vi "UHR-Fleezers Control (host) -Mau_stepping.vi"(0 "Tab Control":T5(tab)) -> ()   [LabVIEW 2013] (continued)
            n684 = local read "Green FB On/Off"() -> (w1119:bool)
            n685 = Equal?(x=w1122, y=enum32{"Laser ON", "Laser OFF", "Interlace"}."Interlace") -> (x = y?=w1120:bool)
            n686 = And(x=w1120, y=w1119) -> (x .and. y?=w1118:bool)
          }
        }
        n687 = xnode "Read/Write Control"("FPGA VI Reference In"=w1115, "error in"=w1113, "Operating Mode"=w1110, "Operating Mode 2"=w1110, "Green FB On/Off"=w1109) -> ("error out"=w1114:errorcluster)  [unwired: 1 out]
      }
      event "- phase (APD 1 Gate)", "+ phase (APD 1 Gate)": Value Change {
        n688 = event-data() -> ()  [unwired: 7 out]
        n689 = local read "Phase Adj. (APD 1 Gate)"() -> (w1123:i16)
        n690 = Negate(x=w1123) -> (-x=w1131:i16)
        n691 = Select(t=w1131, s="- phase (APD 1 Gate)", f=w1123) -> (s? t:f=w1130:i16)
        n692 = Or(x="- phase (APD 1 Gate)", y="+ phase (APD 1 Gate)") -> (x .or. y?=w1126:bool)
        n693 = xnode "Read/Write Control"("FPGA VI Reference In"=w1133, "error in"=w1132, "Phase count adjustment (APD 1 Gate)"=w1130) -> ("FPGA VI Reference Out"=w1128:T19, "error out"=w1129:errorcluster)
        n694 = xnode "Read/Write Control"("FPGA VI Reference In"=w1128, "error in"=w1129, "+ phase (APD 1 Gate)"=w1126) -> ("error out"=w1127:errorcluster)  [unwired: 1 out]
      }
      event "+ phase (APD 2 Gate)", "- phase (APD 2 Gate)": Value Change {
        n695 = event-data() -> ()  [unwired: 7 out]
        n696 = local read "Phase Adj. (APD 2 Gate)"() -> (w1134:i16)
        n697 = Negate(x=w1134) -> (-x=w1142:i16)
        n698 = Select(t=w1142, s="- phase (APD 2 Gate)", f=w1134) -> (s? t:f=w1141:i16)
        n699 = Or(x="- phase (APD 2 Gate)", y="+ phase (APD 2 Gate)") -> (x .or. y?=w1137:bool)
        n700 = xnode "Read/Write Control"("FPGA VI Reference In"=w1144, "error in"=w1143, "Phase count adjustment (APD 2 Gate)"=w1141) -> ("FPGA VI Reference Out"=w1139:T19, "error out"=w1140:errorcluster)
        n701 = xnode "Read/Write Control"("FPGA VI Reference In"=w1139, "error in"=w1140, "+ phase (APD 2 Gate)"=w1137) -> ("error out"=w1138:errorcluster)  [unwired: 1 out]
      }
      event "Phase Adj. (APD Acq)", "+ phase (APD Acq)", "- phase (APD Acq)": Value Change {
        n702 = event-data() -> ()  [unwired: 7 out]
        n703 = local read "Phase Adj. (APD Acq)"() -> (w1147:i16)
        n704 = Negate(x=w1147) -> (-x=w1153:i16)
        n705 = Select(t=w1153, s="+ phase (APD Acq)", f=w1147) -> (s? t:f=w1152:i16)
        n706 = Or(x="+ phase (APD Acq)", y="- phase (APD Acq)") -> (x .or. y?=w1148:bool)
        n707 = xnode "Read/Write Control"("FPGA VI Reference In"=w1155, "error in"=w1154, "Phase Count Adjustment (APD Acq)"=w1152) -> ("FPGA VI Reference Out"=w1150:T19, "error out"=w1151:errorcluster)
        n708 = xnode "Read/Write Control"("FPGA VI Reference In"=w1150, "error in"=w1151, "+ phase (APD Acq)"=w1148) -> ("error out"=w1149:errorcluster)  [unwired: 1 out]
      }
      event "Phase adj. (GI)", "+ phase (GI)", "- phase (GI)": Value Change {
        n709 = event-data() -> ()  [unwired: 7 out]
        n710 = Negate(x="Phase adj. (GI)") -> (-x=w1164:i16)
        n711 = Select(t=w1164, s="+ phase (GI)", f="Phase adj. (GI)") -> (s? t:f=w1163:i16)
        n712 = Or(x="+ phase (GI)", y="- phase (GI)") -> (x .or. y?=w1159:bool)
        n713 = xnode "Read/Write Control"("FPGA VI Reference In"=w1166, "error in"=w1165, "Phase count adjustment (GI)"=w1163) -> ("FPGA VI Reference Out"=w1161:T19, "error out"=w1162:errorcluster)
        n714 = xnode "Read/Write Control"("FPGA VI Reference In"=w1161, "error in"=w1162, "+ phase (GI)"=w1159) -> ("error out"=w1160:errorcluster)  [unwired: 1 out]
      }
      event "Phase adj. (GI) 2", "+ phase (GI) 2", "- phase (GI) 2": Value Change {
        n715 = event-data() -> ()  [unwired: 7 out]
        n716 = Negate(x="Phase adj. (GI) 2") -> (-x=w1175:i16)
        n717 = Select(t=w1175, s="+ phase (GI) 2", f="Phase adj. (GI) 2") -> (s? t:f=w1174:i16)
        n718 = Or(x="+ phase (GI) 2", y="- phase (GI) 2") -> (x .or. y?=w1170:bool)
        n719 = xnode "Read/Write Control"("FPGA VI Reference In"=w1177, "error in"=w1176, "Phase count adjustment (GI) 2"=w1174) -> ("FPGA VI Reference Out"=w1172:T19, "error out"=w1173:errorcluster)
        n720 = xnode "Read/Write Control"("FPGA VI Reference In"=w1172, "error in"=w1173, "+ phase (GI) 2"=w1170) -> ("error out"=w1171:errorcluster)  [unwired: 1 out]
      }
      event "Phase adj. (Green FB)", "- phase (Green FB)", "+ phase (Green FB)": Value Change {
        n721 = event-data() -> ()  [unwired: 7 out]
        n722 = Negate(x="Phase adj. (Green FB)") -> (-x=w1186:i16)
        n723 = Select(t=w1186, s="+ phase (Green FB)", f="Phase adj. (Green FB)") -> (s? t:f=w1185:i16)
        n724 = Or(x="+ phase (Green FB)", y="- phase (Green FB)") -> (x .or. y?=w1181:bool)
        n725 = xnode "Read/Write Control"("FPGA VI Reference In"=w1188, "error in"=w1187, "Phase count adjustment (Green FB)"=w1185) -> ("FPGA VI Reference Out"=w1183:T19, "error out"=w1184:errorcluster)
        n726 = xnode "Read/Write Control"("FPGA VI Reference In"=w1183, "error in"=w1184, "+ phase (Green FB)"=w1181) -> ("error out"=w1182:errorcluster)  [unwired: 1 out]
      }
      event "Invert APD Gate", "APD Gate ON Count", "APD Gate OFF Count", "APD Gate", "APD Integration Time (s)", "APD 1 AO Mult.", "APD 2 AO Mult.": Value Change {
        n727 = event-data() -> ()  [unwired: 7 out]
        n728 = local read "APD Integration Time (s)"() -> (w1189:dbl)
        n729 = local read "APD Gate ON Count"() -> (w1202:u32)
        n730 = local read "APD Gate OFF Count"() -> (w1201:u32)
        n731 = local read "Invert APD Gate"() -> (w1203:bool)
        n732 = local read "APD Gate"() -> (w1200:enum32{"ON", "OFF", "Interlace"})
        n733 = Multiply(x=w1189, y=40000000.0) -> (x*y=w1198:dbl)
        n734 = Reciprocal(x=w1189) -> (1/x=→"APD Acq Rate (Hz)":dbl)
        n735 = To Unsigned Long Integer(number=w1198) -> (unsigned 32bit integer=w1197:u32)
        n736 = local read "DMA Update Period (s)"() -> (w1190:dbl)
        n737 = Divide(x=w1190, y=w1189) -> (x/y=w1193:dbl)
        n738 = local read "APD 1 AO Mult."() -> (w1195:i16)
        n739 = local read "APD 2 AO Mult."() -> (w1194:i16)
        n740 = Multiply(x=2.0, y=w1193) -> (x*y=w1192:dbl)
        n741 = local write "APD Samples/FIFO Acq."(w1193) -> ()
        n742 = local write "APD Elements/DMA read"(w1192) -> ()
        n743 = xnode "Read/Write Control"("FPGA VI Reference In"=w1206, "error in"=w1205, "Invert APD Gate"=w1203, "APD Gate ON Count"=w1202, "APD Gate OFF Count"=w1201, "APD Acq Rate Count"=w1197, "APD Gate Operating Mode"=w1200, "APD 1 AO scale factor"=w1195, "APD 2 AO scale factor"=w1194) -> ("error out"=w1204:errorcluster)  [unwired: 1 out]
      }
      event "GI Frequency, ON count", "Green FB Count", "GI Frequency, OFF count": Value Change {
        n744 = event-data() -> ()  [unwired: 7 out]
        n745 = xnode "Read/Write Control"("FPGA VI Reference In"=w1212, "error in"=w1210, "Green interlace ON count"="GI Frequency, ON count", "Green interlace OFF count"="GI Frequency, OFF count", "Green interlace ON count 2"="GI Frequency, ON count", "Green interlace OFF count 2"="GI Frequency, OFF count", "Green FB Count"="Green FB Count") -> ("error out"=w1211:errorcluster)  [unwired: 1 out]
      }
      event "Number of F/B Scans (AOD)", "Scan Speed (nm/s)", "Scan BD", "Initial delta (MHz)", "Step Size (nm)", "Scan Range (nm)": Value Change {
        w1274 = 123.0  # AOM cal (nm/MHz)
        n746 = event-data() -> ()  [unwired: 7 out]
        n747 = local read "BD 1 Frequency 1 (MHz)"() -> (w1257:dbl)
        n748 = local read "AOM X Cal (nm/MHz)"() -> (w1249:dbl)
        n749 = local read "X RF Frequency Limits (MHz)"() -> (w1261:T16)
        n750 = local read "Y RF Frequency Limits (MHz)"() -> (w1258:T16)
        n751 = local read "BD 2 Frequency 1 (MHz)"() -> (w1263:dbl)
        n752 = Negate(x="Scan Range (nm)") -> (-x=w1227:dbl)
        n753 = Divide(x=w1227, y=w1249) -> (x/y=w1231:dbl)
        n754 = Select(t=w1261, s="Scan BD", f=w1258) -> (s? t:f=w1260:T16)
        n755 = Select(t=w1257, s="Scan BD", f=w1263) -> (s? t:f=w1262:dbl)
        n756 = Unbundle By Name(w1260) -> ("Maximum"=w1269:dbl, "Minimum"=w1268:dbl)
        n757 = Add(x=w1231, y=w1262) -> (x+y=w1266:dbl)
        n758 = Divide(x=w1227, y="Step Size (nm)") -> (x/y=w1246:dbl)
        n759 = Divide(x="Step Size (nm)", y=w1249) -> (x/y=w1255:dbl)
        n760 = Absolute Value(x=w1246) -> (abs(x)=w1230:dbl)
        n761 = Sign(1:w1227) -> (0:w1228:dbl)
        n762 = In Range and Coerce(upper limit=w1269, x=w1266, lower limit=w1268) -> (coerced(x)=w1265:dbl, In Range?=w1267:bool)
        n763 = To Unsigned Quad Integer(1:w1230) -> (0:w1245:u64)
        "Scan steps (AOD)" <- w1245
        n764 = call "IR AOM freq to word.vi"("Frequency In (MHz)"=w1255) -> ("Frequency Word Out (double)"=w1252:dbl)
        n765 = Multiply(x=w1228, y=w1252) -> (x*y=w1229:dbl)
        n766 = Subtract(x=w1266, y=w1265) -> (x-y=w1264:dbl)
        n767 = To Quad Integer(1:w1229) -> (0:w1251:i64)
        "Incr. int (AOD)" <- w1251
        n768 = Subtract(x=w1231, y=w1264) -> (x-y=w1250:dbl)
        "Scan Range (MHz)" <- w1250
        n769 = Select(t=w1231, s=w1267, f=w1250) -> (s? t:f=w1270:dbl)
        n770 = Multiply(x=w1250, y=w1249) -> (x*y=w1248:dbl)
        n771 = Decrement(x=w1245) -> (x-1=w1298:u64)
        n772 = Negate(x=w1248) -> (-x=w1244:dbl)
        n773 = local write "Scan Range (nm)"(w1244) -> ()
        n774 = Divide(x=w1270, y=w1298) -> (x/y=w1254:dbl)
        "Scan Increment (MHz)" <- w1254
        n775 = call "IR AOM freq to word.vi"("Frequency In (MHz)"=w1254) -> ("Frequency Word Out (double)"=w1253:dbl)
        n776 = Divide(x="Step Size (nm)", y="Scan Speed (nm/s)") -> (x/y=w1241:dbl)
        n777 = To Quad Integer(1:w1253) -> ()  [unwired: 1 out]
        n778 = local read "Number Interlace Sets"() -> (w1225:u8)
        n779 = local read "AI Count (ticks)"() -> (w1226:u32)
        n780 = local read "Total Counts (ticks)"() -> (w1224:u32)
        n781 = local read "# Samples/trap"() -> (w1256:u32)
        n782 = Multiply(x=w1226, y=w1225) -> (x*y=w1223:u32)
        n783 = Divide(x=w1224, y=w1223) -> (x/y=w1222:dbl)
        n784 = Select(t=w1257, s="Scan BD", f=w1263) -> (s? t:f=w1295:dbl)
        "Initial freq. (MHz)" <- w1295
        n785 = Add(x=w1270, y=w1295) -> (x+y=→"Final freq. (MHz)":dbl)
        n786 = Divide(x=w1224, y=40000000.0) -> (x/y=w1240:dbl)
        n787 = Divide(x=w1241, y=w1240) -> (x/y=w1239:dbl)
        n788 = To Unsigned Quad Integer(1:w1239) -> (0:w1214:u64)
        n789 = Quotient & Remainder(x=w1214, y=u64 2) -> (x-y*floor(x/y)=w1218:u64)  [unwired: 1 out]
        n790 = Equal?(x=w1218, y=u64 0) -> (x = y?=w1216:bool)
        n791 = Decrement(x=w1214) -> (x-1=w1215:u64)
        n792 = Select(t=w1214, s=w1216, f=w1215) -> (s? t:f=w1213:u64)
        "Cycles/step (AOD)" <- w1213
        n793 = xnode "Read/Write Control"("FPGA VI Reference In"=w1306, "error in"=w1305, "Scan steps"=w1245, "Number of scans"="Number of F/B Scans (AOD)", "Cycles per step"=w1213, "Scan freq.  increment"=w1251, "Scan BD"="Scan BD") -> ("error out"=w1304:errorcluster)  [unwired: 1 out]
        n794 = Multiply(x=w1245, y=w1213) -> (x*y=w1299:u64)
        n795 = Multiply(x=w1299, y=u64 2) -> (x*y=w1221:u64)
        n796 = Multiply(x=w1222, y=w1221) -> (x*y=w1220:dbl)
        "Data points/scan (f/b)" <- w1220
        n797 = Multiply(x=w1220, y="Number of F/B Scans (AOD)") -> (x*y=w1302:dbl)
        "Data points/scans" <- w1302
        n798 = Divide(x=w1302, y=w1256) -> (x/y=→"N sets should be saved":dbl)
        n799 = Multiply(x=w1299, y=w1240) -> (x*y=w1238:dbl)
        "Time/Scan (s) (AOD)" <- w1238
        n800 = Select(t=w1270, s="Scan BD", f=0.0) -> (s? t:f=w1296:dbl)
        n801 = Select(t=0.0, s="Scan BD", f=w1270) -> (s? t:f=w1292:dbl)
        n802 = local read "BD 2 Frequency 2 (MHz)"() -> (w1288:dbl)
        n803 = local read "BD 1 Frequency 2 (MHz)"() -> (w1291:dbl)
        n804 = Add(x=w1292, y=w1263) -> (x+y=w1289:dbl)
        n805 = Add(x=w1257, y=w1296) -> (x+y=w1290:dbl)
        n806 = Multiply(x=w1238, y=2.0) -> (x*y=w1237:dbl)
        n807 = Multiply(x=w1237, y="Number of F/B Scans (AOD)") -> (x*y=w1234:dbl)
        n808 = Divide(x=w1234, y=60.0) -> (x/y=→"Time to Finish All (min)":dbl)
        n809 = Add(x="Trap 2 Bead Size (nm)", y="Trap 1 Bead Size (nm)") -> (x+y=w1278:dbl)
        n810 = local read "Initial delta (MHz)"() -> (w1275:dbl)
        n811 = Divide(x=w1278, y=2.0) -> (x/y=w1272:dbl)
        n812 = Subtract(x=w1289, y=w1288) -> (x-y=w1286:dbl)
        n813 = Subtract(x=w1290, y=w1291) -> (x-y=w1287:dbl)
        n814 = Square(x=w1286) -> (x^2=w1285:dbl)
        n815 = Square(x=w1287) -> (x^2=w1284:dbl)
        n816 = Add(x=w1284, y=w1285) -> (x+y=w1283:dbl)
        n817 = Square Root(x=w1283) -> (sqrt(x)=w1282:dbl)
        "Final delta (MHz)" <- w1282
        n818 = Multiply(x=w1274, y=w1282) -> (x*y=w1281:dbl)
        n819 = Multiply(x=w1275, y=w1274) -> (x*y=w1273:dbl)
        n820 = Subtract(x=w1273, y=w1272) -> (x-y=→"Initial sep (nm)":dbl)
        n821 = Subtract(x=w1281, y=w1272) -> (x-y=→"Final sep (nm)":dbl)
      }
      event "Raster Scanning...": Value Change {
        n822 = event-data() -> ("NewVal"=w1307:bool)  [unwired: 6 out]
        n823 = case shown="True" w1307 {
          frame False {
          }
          frame True {
            n824 = property on="BD 1 Frequency 1 (MHz)" class="DigNum (strict)"("Val(Sgnl)"=65.0 ("Value (Signaling)")) -> ()  [unwired: 2 in, 2 out]
          }
        }
      }
      event "Freq or Amp switch first", "Swap F1 and F2", "Freq switch delay", "Amp switch delay": Value Change {
        n825 = event-data() -> ()  [unwired: 7 out]
        n826 = local read "Freq or Amp switch first"() -> (w1309:bool)
        n827 = local read "Amp switch delay"() -> (w1310:u16)
        n828 = local read "Freq switch delay"() -> (w1312:u16)
        n829 = local read "Swap F1 and F2"() -> (w1311:bool)
        n830 = xnode "Read/Write Control"("FPGA VI Reference In"=w1315, "error in"=w1314, "Freq switch delay"=w1312, "Swap F1 and F2"=w1311, "Amp switch delay"=w1310, "Freq or Amp switch first"=w1309) -> ("error out"=w1313:errorcluster)  [unwired: 1 out]
      }
      event "Scan steps (MCL)", "Number of scans (MCL)", "Scan Range (V)\n(of steps)", "2D or 1D Scan", "N APD Samp/step", "Fast Scan Dir", "Continuous MCL Scanning", "Scan lines (y)": Value Change {
        w1317 = 32767.0 ("y")
        n831 = event-data() -> ()  [unwired: 7 out]
        n832 = Select(t="Scan lines (y)", s="2D or 1D Scan", f="Number of scans (MCL)") -> (s? t:f=w1322:u64)
        n833 = Decrement(x="Scan steps (MCL)") -> (x-1=w1338:u64)
        n834 = Divide(x="Scan Range (V)\n(of steps)", y=w1338) -> (x/y=w1337:dbl)
        "Desired Scan Incr (V)" <- w1337
        n835 = local read "APD Integration Time (s)"() -> (w1330:dbl)
        n836 = Multiply(x=w1337, y=w1317) -> (x*y=w1346:dbl)
        n837 = Divide(x=w1346, y=10.0) -> (x/y=w1336:dbl)
        "Desired incr (int)" <- w1336
        n838 = local read "Update Count (MCL)"() -> (w1342:u32)
        n839 = Round Toward -Infinity(1:w1336) -> (0:w1345:dbl)
        n840 = To Word Integer(number=w1345) -> (16bit integer=w1320:i16)
        "Actual Incr. int (MCL)" <- w1320
        n841 = Multiply(x=w1330, y=40000000.0) -> (x*y=w1343:dbl)
        n842 = Divide(x=w1343, y=w1342) -> (x/y=w1341:dbl)
        n843 = Multiply(x=i16 10, y=w1320) -> (x*y=w1318:i16)
        n844 = Multiply(x="N APD Samp/step", y=w1341) -> (x*y=w1340:dbl)
        "Cycles/step (MCL)" <- w1340
        n845 = Divide(x=w1318, y=w1317) -> (x/y=→"Actual MCL Inc (V)":dbl)
        n846 = Multiply(x="N APD Samp/step", y="Scan steps (MCL)") -> (x*y=w1332:dbl)
        n847 = local read "APD Samples/FIFO Acq."() -> (w1329:dbl)
        n848 = Multiply(x=w1332, y=u64 2) -> (x*y=w1331:dbl)
        "Data points/scan (f+b)" <- w1331
        n849 = Multiply(x=w1331, y=w1322) -> (x*y=w1349:dbl)
        "Data points/scans (MCL)" <- w1349
        n850 = Multiply(x=w1330, y=w1331) -> (x*y=w1323:dbl)
        "Time/f+b scan (s) (MCL)" <- w1323
        n851 = Divide(x=w1349, y=w1329) -> (x/y=→"N sets should be saved (MCL)":dbl)
        n852 = Multiply(x=w1323, y=w1322) -> (x*y=→"Total Time (s)":dbl)
        n853 = Not(x="Fast Scan Dir") -> (.not. x?=w1327:bool)
        n854 = xnode "Read/Write Control"("FPGA VI Reference In"=w1353, "error in"=w1352, "Scan steps (MCL)"="Scan steps (MCL)", "Number of scans (MCL)"=w1322, "Cycles per step (MCL)"=w1340, "Scan freq.  increment (MCL)"=w1320, "1D or 2D Scan?"="2D or 1D Scan", "MCL Scan Axis"=w1327, "Cont. Scan (MCL)"="Continuous MCL Scanning") -> ("error out"=w1351:errorcluster)  [unwired: 1 out]
      }
      event "Read Cal": Value Change {
        w1355 = 1000.0 ("y")
        n855 = event-data() -> ()  [unwired: 7 out]
        n856 = local read "Save file name"() -> (w1380:path)
        n857 = local write "Read Cal"(FALSE ("Read Cal")) -> ()
        n858 = Strip Path(path=w1380) -> (stripped path=w1379:path)  [unwired: 1 out]
        n859 = Path To String(path=w1379) -> (string=w1378:string)
        n860 = Concatenate Strings(w1378, "\\current.cal" ("string")) -> (w1376:string)
        n861 = String To Path(string=w1376) -> (path=w1375:path)
        n862 = Open/Create/Replace File(file path (use dialog)=w1375, operation (0:open)=T23."open", access (0:read/write)=enum16{"read/write", "read-only", "write-only"}."read-only") -> (refnum out=w1383:refnum<file>, error out=w1369:errorcluster)  [unwired: 1 in, 3 out]
        n863 = Deny Access(4:w1369, 7:w1383) -> (0:w1368:errorcluster, 3:w1374:refnum<file>)  [unwired: 1 out]
        n864 = Read from Binary File(5:0.0, 8:w1368, 9:T29."big-endian, network order" ("byte order (0:big-endian, network order)"), 10:-1 ("count (1)"), 11:w1374) -> (0:w1367:errorcluster, 2:w1365:dbl[], 3:w1370:refnum<file>)  [unwired: 2 out]
        n865 = Array To Cluster(array=w1365) -> (cluster=w1364:T31)
        n866 = Unbundle(w1364) -> ("[0]"=w1363:dbl, "[1]"=w1362:dbl, "[2]"=w1361:dbl, "[3]"=w1360:dbl, "[4]"=w1359:dbl, "[5]"=w1358:dbl)
        n867 = Close File(refnum=w1370, error in=w1367) -> (error out=→"Read cal error":errorcluster)  [unwired: 1 out]
        n868 = Multiply(x=w1358, y=w1355) -> (x*y=w1356:dbl)
        n869 = local write "T2 kappa_x (pN/nm)"(w1360) -> ()
        n870 = local write "T1 kappa_x (pN/nm)"(w1361) -> ()
        n871 = local write "T1 alpha_x (nm/V)"(w1363) -> ()
        n872 = local write "T2 alpha_x (nm/V)"(w1362) -> ()
        n873 = Multiply(x=w1359, y=w1355) -> (x*y=w1357:dbl)
        n874 = local write "T1 offset_x (mV)"(w1357) -> ()
        n875 = local write "T2 offset_x (mV)"(w1356) -> ()
      }
      event "Abort MCL Scan": Value Change {
        n876 = event-data() -> ()  [unwired: 7 out]
        n877 = local write "MCL Scanning"(FALSE ("MCL Scanning")) -> ()
        n878 = xnode "Read/Write Control"("FPGA VI Reference In"=w1388, "error in"=w1387, "Abort scan (MCL)"="Abort MCL Scan") -> ("error out"=w1386:errorcluster)  [unwired: 1 out]
      }
      event "Update Count (MCL)": Value Change {
        n879 = event-data() -> ()  [unwired: 7 out]
        n880 = xnode "Read/Write Control"("FPGA VI Reference In"=w1392, "error in"=w1391, "MCL count"="Update Count (MCL)") -> ("error out"=w1390:errorcluster)  [unwired: 1 out]
      }
      event "Phase adjust (MCL)", "+ phase (MCL)", "- phase (MCL)": Value Change {
        n881 = event-data() -> ()  [unwired: 7 out]
        n882 = Negate(x="Phase adjust (MCL)") -> (-x=w1401:i16)
        n883 = Select(t=w1401, s="- phase (MCL)", f="Phase adjust (MCL)") -> (s? t:f=w1399:i16)
        n884 = Or(x="- phase (MCL)", y="+ phase (MCL)") -> (x .or. y?=w1394:bool)
        n885 = xnode "Read/Write Control"("FPGA VI Reference In"=w1403, "error in"=w1402, "Phase count adjustment (MCL)"=w1399) -> ("FPGA VI Reference Out"=w1395:T19, "error out"=w1396:errorcluster)
        n886 = xnode "Read/Write Control"("FPGA VI Reference In"=w1395, "error in"=w1396, "+ phase (MCL)"=w1394) -> ("error out"=w1393:errorcluster)  [unwired: 1 out]
      }
      event "Abort AOD Scan": Value Change {
        n887 = event-data() -> ()  [unwired: 7 out]
        n888 = xnode "Read/Write Control"("FPGA VI Reference In"=w1407, "error in"=w1406, "Abort scan"="Abort AOD Scan") -> ("error out"=w1405:errorcluster)  [unwired: 1 out]
      }
      event "Continuous AOD Scanning": Value Change {
        n889 = event-data() -> ()  [unwired: 7 out]
        n890 = xnode "Read/Write Control"("FPGA VI Reference In"=w1411, "error in"=w1410, "Cont. Scan"="Continuous AOD Scanning") -> ("error out"=w1409:errorcluster)  [unwired: 1 out]
      }
      event "Index": Value Change {
        n891 = event-data() -> ()  [unwired: 7 out]
        n892 = call "Create new save file.vi"("Insert"="", "Ext"=".dat" ("string"), "Index In"="Index") -> ("Path Out"=→"Save file name":path, "Index Out"=w1412:dbl)
        "Save index" <- w1412
        n893 = local write "Index"(w1412) -> ()
      }
      event "AO1", "AO2": Value Change {
        w1427 = 10.0 ("y")
        w1426 = 32767.0 ("y")
        n894 = event-data() -> ()  [unwired: 7 out]
        n895 = local read "AO2"() -> (w1425:dbl)
        n896 = local read "AO1"() -> (w1422:dbl)
        n897 = Multiply(x=w1422, y=w1426) -> (x*y=w1421:dbl)
        n898 = Multiply(x=w1425, y=w1426) -> (x*y=w1424:dbl)
        n899 = Divide(x=w1421, y=w1427) -> (x/y=w1420:dbl)
        n900 = Divide(x=w1424, y=w1427) -> (x/y=w1423:dbl)
        n901 = To Word Integer(number=w1420) -> (16bit integer=w1428:i16)
        n902 = To Word Integer(number=w1423) -> (16bit integer=w1429:i16)
        n903 = xnode "Read/Write Control"("FPGA VI Reference In"=w1419, "error in"=w1418, "AO1"=w1428, "AO2"=w1429) -> ("error out"=w1417:errorcluster)  [unwired: 1 out]
      }
      event "Inject Top:": Value Change {
        n904 = event-data() -> ()  [unwired: 7 out]
        n905 = disable-structure shown="Enabled" {
          disable-tunnel: "Inject Top:" -> [w1431 w1471]
          frame Disabled {
            n906 = local read "Chemyx Syringe Pump Serial Port"() -> (w1432:refnum<visa-resource-name>)
            n907 = local read "Pump write delay (ms)"() -> (w1433:dbl)
            n908 = case shown="True" w1431 {
              tunnel: w1433 -> [w1439 w1453]
              tunnel: w1432 -> [w1436 w1452]
              frame False {
                n909 = flat-sequence {
                  tunnel: w1436 -> [w1440]
                  tunnel: [w1440] -> w1437
                  tunnel: w1439 -> [_]
                  tunnel: [w1443] -> w1438
                  tunnel: w1437 -> [w1443]
                  tunnel: w1438 -> [w1444]
                  tunnel: [w1444] -> w1434
                  tunnel: [w1446] -> w1435
                  tunnel: w1434 -> [w1446]
                  tunnel: w1435 -> [w1448]
                  frame #0 {
                    n910 = call "Write to pump.vi"("string"="enter pump1", "VISA resource name"=w1440) -> ()  [unwired: 1 out]
                  }
                  frame #1 {
                    n911 = Wait (ms)(milliseconds to wait="Pump pause delay (ms)") -> ()  [unwired: 1 out]
                  }
                  frame #2 {
                    n912 = call "Write to pump.vi"("string"="stop", "VISA resource name"=w1444) -> ()  [unwired: 1 out]
                  }
                  frame #3 {
                    n913 = Wait (ms)(milliseconds to wait=u32 500) -> ()  [unwired: 1 out]
                  }
                  frame #4 {
                    n914 = call "Write to pump.vi"("string"="stop", "VISA resource name"=w1448) -> ()  [unwired: 1 out]
                  }
                }
              }
              frame True {
                n915 = flat-sequence {
                  tunnel: w1452 -> [w1462]
                  tunnel: w1453 -> [w1457]
                  tunnel: w1453 -> [w1464]
                  tunnel: w1452 -> [w1465]
                  tunnel: [w1465] -> w1450
                  tunnel: [w1467] -> w1451
                  tunnel: w1450 -> [w1467]
                  tunnel: w1451 -> [w1469]
                  frame #0 {
                    n916 = local read "All Pump Parameters"() -> (w1456:T6)
                    n917 = Unbundle By Name(w1456) -> ("Pump 1"=w1463:T32)
                    n918 = call "Set pump parameters.vi"("Pump write delay (ms)"=w1457, "Volume (uL)"="Ch 2 Inject Volume (uL)", "Rate (uL/h)"="Ch 1 Inject Rate (ul/h)", "Units"=4.0, "Pump #"=1.0, "Pump Parameters In"=w1463, "VISA resource name"=w1462) -> ("Pump Parameters Out"=w1455:T32)  [unwired: 3 in]
                    n919 = Bundle By Name(cluster=w1456, "Pump 1"=w1455) -> (w1454:T6)
                    n920 = local write "All Pump Parameters"(w1454) -> ()
                  }
                  frame #1 {
                    n921 = Wait (ms)(milliseconds to wait=w1464) -> ()  [unwired: 1 out]
                  }
                  frame #2 {
                    n922 = call "Write to pump.vi"("string"="start", "VISA resource name"=w1465) -> ()  [unwired: 1 out]
                  }
                  frame #3 {
                    n923 = Wait (ms)(milliseconds to wait=u32 500) -> ()  [unwired: 1 out]
                  }
                  frame #4 {
                    n924 = call "Write to pump.vi"("string"="start", "VISA resource name"=w1469) -> ()  [unwired: 1 out]
                  }
                }
              }
            }
          }
          frame Enabled {
            n925 = call "hamilton_controller.vi"("Open?"=w1471, "valve"=enum16{"A", "B", "C", "D", "ALL"}."B", "action"=T20."MOVE VALVE") -> ()  [unwired: 8 in, 1 out]
          }
        }
      }
      event "Main:": Value Change {
        n926 = event-data() -> ()  [unwired: 7 out]
        n927 = disable-structure shown="Disabled" {
          disable-tunnel: "Main:" -> [_ w1515]
          frame Disabled {
            n928 = local read "Pump write delay (ms)"() -> (w1476:dbl)
            n929 = case shown="False" w1477 {
              tunnel: w1476 -> [w1483 w1497]
              tunnel: "Chemyx Syringe Pump Serial Port" -> [w1480 w1496]
              frame False {
                n930 = flat-sequence {
                  tunnel: w1480 -> [w1484]
                  tunnel: [w1484] -> w1481
                  tunnel: w1483 -> [_]
                  tunnel: [w1487] -> w1482
                  tunnel: w1481 -> [w1487]
                  tunnel: w1482 -> [w1488]
                  tunnel: [w1488] -> w1478
                  tunnel: [w1490] -> w1479
                  tunnel: w1478 -> [w1490]
                  tunnel: w1479 -> [w1492]
                  frame #0 {
                    n931 = call "Write to pump.vi"("string"="enter pump3", "VISA resource name"=w1484) -> ()  [unwired: 1 out]
                  }
                  frame #1 {
                    n932 = local read "Pump pause delay (ms)"() -> (w1486:u32)
                    n933 = Wait (ms)(milliseconds to wait=w1486) -> ()  [unwired: 1 out]
                  }
                  frame #2 {
                    n934 = call "Write to pump.vi"("string"="stop", "VISA resource name"=w1488) -> ()  [unwired: 1 out]
                  }
                  frame #3 {
                    n935 = Wait (ms)(milliseconds to wait=u32 0) -> ()  [unwired: 1 out]
                  }
                  frame #4 {
                    n936 = call "Write to pump.vi"("string"="stop", "VISA resource name"=w1492) -> ()  [unwired: 1 out]
                  }
                }
              }
              frame True {
                n937 = flat-sequence {
                  tunnel: w1496 -> [w1506]
                  tunnel: w1497 -> [w1501]
                  tunnel: w1497 -> [w1508]
                  tunnel: w1496 -> [w1509]
                  tunnel: [w1509] -> w1494
                  tunnel: [w1512] -> w1495
                  tunnel: w1494 -> [w1512]
                  tunnel: w1495 -> [w1513]
                  frame #0 {
                    n938 = local read "All Pump Parameters"() -> (w1500:T6)
                    n939 = Unbundle By Name(w1500) -> ("Pump 3"=w1507:T32)
                    n940 = call "Set pump parameters.vi"("Pump write delay (ms)"=w1501, "Volume (uL)"="Ch 3 Inject Volume (uL)", "Rate (uL/h)"="Ch 3 Inject Rate (ul/h)", "Units"=4.0, "Pump #"=3.0, "Pump Parameters In"=w1507, "VISA resource name"=w1506) -> ("Pump Parameters Out"=w1499:T32)  [unwired: 3 in]
                    n941 = Bundle By Name(cluster=w1500, "Pump 3"=w1499) -> (w1498:T6)
                    n942 = local write "All Pump Parameters"(w1498) -> ()
                  }
                  frame #1 {
                    n943 = Wait (ms)(milliseconds to wait=w1508) -> ()  [unwired: 1 out]
                  }
                  frame #2 {
                    n944 = call "Write to pump.vi"("string"="start", "VISA resource name"=w1509) -> ()  [unwired: 1 out]
                  }
                  frame #3 {
                    n945 = Wait (ms)(milliseconds to wait=u32 500) -> ()  [unwired: 1 out]
                  }
                  frame #4 {
                    n946 = call "Write to pump.vi"("string"="start", "VISA resource name"=w1513) -> ()  [unwired: 1 out]
                  }
                }
              }
            }
          }
          frame Enabled {
            n947 = call "hamilton_controller.vi"("Open?"=w1515, "valve"=enum16{"A", "B", "C", "D", "ALL"}."A", "action"=T20."MOVE VALVE") -> ()  [unwired: 8 in, 1 out]
          }
        }
      }
      event "Inject Valve B": Value Change {
        n948 = event-data() -> ()  [unwired: 7 out]
        n949 = disable-structure shown="Enabled" {
          disable-tunnel: "Inject Valve B" -> [w1519 w1539]
          frame Disabled {
            n950 = local read "Pump write delay (ms)"() -> (w1521:dbl)
            n951 = flat-sequence {
              tunnel: w1520 -> [w1534]
              tunnel: w1521 -> [w1530]
              tunnel: w1519 -> [_]
              tunnel: w1521 -> [w1536]
              tunnel: w1520 -> [w1537]
              frame #0 {
                n952 = local read "All Pump Parameters"() -> (w1529:T6)
                n953 = Multiply(x=60.0, y="Flush Center Ch Rate (ul/m)") -> (x*y=w1526:dbl)
                n954 = Unbundle By Name(w1529) -> ("Pump 2"=w1535:T32)
                n955 = call "Set pump parameters.vi"("Pump write delay (ms)"=w1530, "Volume (uL)"="Flush Center Ch Volume (uL)", "Rate (uL/h)"=w1526, "Units"=3.0, "Pump #"=2.0, "Pump Parameters In"=w1535, "VISA resource name"=w1534) -> ("Pump Parameters Out"=w1528:T32)  [unwired: 3 in]
                n956 = Bundle By Name(cluster=w1529, "Pump 2"=w1528) -> (w1527:T6)
                n957 = local write "All Pump Parameters"(w1527) -> ()
                n958 = Add(x="Flush Center Ch Volume (uL)", y="Total Volume\nFlushed (uL)") -> (x+y=w1523:dbl)
                n959 = local write "Total Volume\nFlushed (uL)"(w1523) -> ()
              }
              frame #1 {
                n960 = Wait (ms)(milliseconds to wait=w1536) -> ()  [unwired: 1 out]
              }
              frame #2 {
                n961 = call "Write to pump.vi"("string"="start", "VISA resource name"=w1537) -> ()  [unwired: 1 out]
              }
            }
            n962 = local read "Chemyx Syringe Pump Serial Port"() -> (w1520:refnum<visa-resource-name>)
          }
          frame Enabled {
            n963 = call "hamilton_controller.vi"("Open?"=w1539, "valve"=enum16{"A", "B", "C", "D", "ALL"}."B", "action"=T20."MOVE VALVE") -> ()  [unwired: 8 in, 1 out]
          }
        }
      }
      event "Inject Bottom": Value Change {
        n964 = event-data() -> ()  [unwired: 7 out]
        n965 = call "hamilton_controller.vi"("Open?"="Inject Bottom", "valve"=enum16{"A", "B", "C", "D", "ALL"}."C", "action"=T20."MOVE VALVE") -> ()  [unwired: 8 in, 1 out]
      }
      event "Shunt:": Value Change {
        n966 = event-data() -> ()  [unwired: 7 out]
        n967 = call "hamilton_controller.vi"("Open?"="Shunt:", "valve"=enum16{"A", "B", "C", "D", "ALL"}."D", "action"=T20."MOVE VALVE") -> ()  [unwired: 8 in, 1 out]
      }
      event "Flip Green Filter": Value Change {
        n968 = event-data() -> ()  [unwired: 7 out]
        n969 = local write "Flip Green Filter"("Flip Green Filter") -> ()
        n970 = flat-sequence {
          tunnel: w1555 -> [w1560]
          tunnel: w1554 -> [w1559]
          tunnel: [w1557] -> w1552
          tunnel: [w1556] -> w1551
          tunnel: [w1562] -> w1550
          tunnel: w1552 -> [w1562]
          tunnel: [w1561] -> w1549
          tunnel: w1551 -> [w1561]
          tunnel: w1550 -> [w1566]
          tunnel: w1549 -> [w1565]
          tunnel: [w1564] -> w1553
          frame #0 {
            n971 = xnode "Read/Write Control"("FPGA VI Reference In"=w1560, "error in"=w1559, "Green Filter Flipper"=TRUE) -> ("FPGA VI Reference Out"=w1557:T19, "error out"=w1556:errorcluster)
          }
          frame #1 {
            n972 = Wait (ms)(milliseconds to wait=u32 100) -> ()  [unwired: 1 out]
          }
          frame #2 {
            n973 = xnode "Read/Write Control"("FPGA VI Reference In"=w1566, "error in"=w1565, "Green Filter Flipper"=FALSE) -> ("error out"=w1564:errorcluster)  [unwired: 1 out]
          }
        }
      }
      event "Pump 1 contents", "Pump 3 contents": Value Change {
        n974 = event-data() -> ()  [unwired: 7 out]
        n975 = local read "Pump 1 contents"() -> (→"Pump 1 cont disp":string)
        n976 = local read "Pump 3 contents"() -> (→"Pump 3 cont disp":string)
      }
      event "Reset Trap Pos. FB": Value Change {
        n977 = event-data() -> ()  [unwired: 7 out]
        n978 = xnode "Read/Write Control"("FPGA VI Reference In"=w1572, "error in"=w1571, "Trap Pos. FB Reset"="Reset Trap Pos. FB") -> ()  [unwired: 2 out]
      }
      event "Trap Pos. FB ON": Value Change {
        n979 = event-data() -> ()  [unwired: 7 out]
        n980 = xnode "Read/Write Control"("FPGA VI Reference In"=w1575, "error in"=w1574, "Force feedback"="Trap Pos. FB ON") -> ()  [unwired: 2 out]
      }
      event "Trap Pos. FB Range", "Trap Pos. FB Gains", "Trap Pos. FB Mult Factor", "Trap Pos. FB Offset Factor", "Trap Pos FB Negate Action", "Trap Pos FB Monitor\nT1 or T2": Value Change {
        n981 = event-data() -> ()  [unwired: 7 out]
        n982 = xnode "Read/Write Control"("FPGA VI Reference In"=w1584, "error in"=w1583, "Trap Pos. FB Range"="Trap Pos. FB Range", "Trap Pos. FB Gains"="Trap Pos. FB Gains", "Trap Pos. FB Mult Factor"="Trap Pos. FB Mult Factor", "Trap Pos. FB Offset Factor"="Trap Pos. FB Offset Factor", "Trap Pos FB Negate Action"="Trap Pos FB Negate Action", "Trap Pos FB Monitor T1 or T2"="Trap Pos FB Monitor\nT1 or T2", "AI1 X Scale"="Trap Pos. AI1 X Pre-scale") -> ()  [unwired: 2 out]
      }
      event "Trap Pos FB SP": Value Change {
        n983 = event-data() -> ()  [unwired: 7 out]
        n984 = xnode "Read/Write Control"("FPGA VI Reference In"=w1587, "error in"=w1586, "Trap Pos. FB SP"="Trap Pos FB SP") -> ()  [unwired: 2 out]
      }
      event "Set SP to Reading": Value Change {
        n985 = event-data() -> ()  [unwired: 7 out]
        n986 = local read "Trap Pos FB Monitor\nT1 or T2"() -> (w1595:bool)
        n987 = local read "Trap X AI1 (DMA)"() -> (w1598:T13)
        n988 = local read "Trap X (AI1)"() -> (w1601:T1)
        n989 = Unbundle By Name(w1601) -> ("Trap 1"=w1600:fxp<+/-,16,1>, "Trap 2"=w1599:fxp<+/-,16,1>)
        n990 = Unbundle By Name(w1598) -> ("Set 1"=w1597:fxp<+/-,16,1>, "Set 2"=w1596:fxp<+/-,16,1>)
        n991 = Select(t=w1600, s=w1595, f=w1599) -> (s? t:f=w1594:fxp<+/-,16,1>)
        n992 = Select(t=w1597, s=w1595, f=w1596) -> (s? t:f=w1593:fxp<+/-,16,1>)
        n993 = Not(x="Set SP Using...") -> (.not. x?=w1588:bool)
        n994 = Select(t=w1594, s=w1588, f=w1593) -> (s? t:f=w1589:fxp<+/-,16,1>)
        n995 = xnode "Read/Write Control"("FPGA VI Reference In"=w1591, "error in"=w1590, "Trap Pos. FB SP"=w1589) -> ()  [unwired: 2 out]
        n996 = local write "Trap Pos FB SP"(w1589) -> ()
      }
      event "Trap Pos. FB Out Scale 2^n": Value Change {
        n997 = event-data() -> ()  [unwired: 7 out]
        n998 = Scale By Power Of 2(n="Trap Pos. FB Out Scale 2^n", x=ext 1.0) -> (x*2^n=w1603:ext)
        n999 = property on="Trap Pos. FB Mult Factor" class="DigNum (strict)"("Val(Sgnl)"=w1603) -> ()  [unwired: 2 in, 2 out]
      }
      event "Trap Pos FB Int Count": Value Change {
        n1000 = event-data() -> ()  [unwired: 7 out]
        n1001 = xnode "Read/Write Control"("FPGA VI Reference In"=w1608, "error in"=w1607, "Trap Pos FB Int Count"="Trap Pos FB Int Count") -> ()  [unwired: 2 out]
      }
    }
    "error out 2" <- w736
    n1002 = node-c288() -> ()  [unwired: 1 in, 1 out]
  }
  n1003 = timed-loop "Run Scripts, including: stage motion" {
    timing: w69 -> [_]
    timing-out: [_] -> w68
    tunnel: w24 -> [_]
    stop <- w1610 stop-if-true
    n1004 = node-c288() -> ()  [unwired: 1 in, 1 out]
    n1005 = event shown="[6] \"Got ADig bead\": Value Change" {
      selector: _ -> [_ _ _ _ _ _ _ _ _ _ _ _]
      dyn-events: _ -> [_ _ _ _ _ _ _ _ _ _ _ _]
      timeout: 50 -> [_ _ _ _ _ _ _ _ _ _ _ _]
      tunnel: ["Move Cap. 1 (DNA Top)" _ "Cal/Data Acq. Spot" "Dump Beads" "Dip for Protein" _ "Got ADig bead" "Got DNA bead" "Take Stepping Data" _ "Take Detection Laser\nImage" _] -> _
      tunnel: [_ _ _ _ _ _ _ _ _ _ _ w1818] -> w1610
      event "Move Cap. 1 (DNA Top)": Value Change {
        n1006 = event-data() -> ()  [unwired: 1 in, 5 out]
        n1007 = local write "Move Cap. 1 (DNA Top)"(FALSE ("Move Cap. 1 (DNA Right)")) -> ()
        n1008 = flat-sequence {
          tunnel: "Cap 1 Samp Flow ON" -> [w1616]
          frame #0 {
            n1009 = local write "Stage Moving"(FALSE ("Stage Moving")) -> ()
            n1010 = case "stop flow" shown="True" w1616 {
              frame False {
              }
              frame True {
                n1011 = call "hamilton_controller.vi"("Open?"=FALSE, "valve"=enum16{"A", "B", "C", "D", "ALL"}."C", "action"=T20."MOVE VALVE") -> ()  [unwired: 8 in, 1 out]
              }
            }
            n1012 = case shown="True" TRUE {
              tunnel: "Cap 1 T ON" -> [w1625 w1626]
              frame False {
                n1013 = property on="Trap 1 (ON/OFF)" class="Bool (strict)"("Val(Sgnl)"=w1625) -> ()  [unwired: 2 in, 2 out]
              }
              frame True {
                n1014 = property on="Trap 2 (ON/OFF)" class="Bool (strict)"("Val(Sgnl)"=w1626) -> ()  [unwired: 2 in, 2 out]
              }
            }
            n1015 = call <vilib>:"Beep.vi"() -> ()  [unwired: 3 in, 9 out]
            n1016 = case shown="True" "Cap 1 Flow ON" {
              frame False {
              }
              frame True {
                n1017 = property on="Main:" class="Bool (strict)"("Val(Sgnl)"=TRUE ("Value (Signaling)")) -> ()  [unwired: 2 in, 2 out]
              }
            }
          }
        }
      }
      event Timeout {
        n1018 = event-data() -> ()  [unwired: 1 in, 2 out]
      }
      event "Cal/Data Acq. Spot": Value Change {
        # "wait for calibration file\nto be written"
        # "signal save cal true\nthis tells the data \nacquisition loop to\nstart sending the data\nto a calibration file"
        # "separate traps to\nthe desired trap delta"
        # "move stage to data acquisition spot"
        # "CHANGE FISH FOR TETHER BACK\nTO TRUE VALUE HERE."
        n1019 = event-data() -> ()  [unwired: 1 in, 5 out]
        n1020 = local write "Cal/Data Acq. Spot"(FALSE ("Cal/Data Acq. Spot")) -> ()
        n1021 = flat-sequence {
          tunnel: ["Cal @ (MHz)"] -> w1627
          tunnel: w1627 -> [w1637]
          tunnel: w1627 -> [w1658]
          frame #0 {
            n1022 = property on="Trap Delta (MHz)" class="DigNum (strict)"("Val(Sgnl)"="Cal @ (MHz)") -> ()  [unwired: 2 in, 2 out]
            n1023 = call <vilib>:"Beep.vi"() -> ()  [unwired: 3 in, 9 out]
          }
          frame #1 {
            n1024 = Wait (ms)(milliseconds to wait=u32 100) -> ()  [unwired: 1 out]
          }
          frame #2 {
            n1025 = property on="Save Calibration" class="Bool (strict)"("Val(Sgnl)"=TRUE ("Value (Signaling)")) -> ()  [unwired: 2 in, 2 out]
          }
          frame #3 {
            n1026 = Wait (ms)(milliseconds to wait=u32 4000) -> ()  [unwired: 1 out]
          }
          frame #4 {
            n1027 = while {
              stop <- w1634 stop-if-true
              n1028 = local read "Saving..."() -> (w1635:bool)
              n1029 = Wait (ms)(milliseconds to wait=u32 100) -> ()  [unwired: 1 out]
              n1030 = Not(x=w1635) -> (.not. x?=w1634:bool)
            }
          }
          frame #5 {
            n1031 = case shown="True" "W/ Offset 1" {
              tunnel: w1637 -> [_ w1639]
              frame False {
              }
              frame True {
                n1032 = stacked-sequence {
                  tunnel: w1639 -> [_ _ _ _ _ _ _ w1656]
                  frame #0 {
                    n1033 = Replace Array Subset(array=u32[] [0] ("Index Values"), new element="Offset 1 Set", index=0) -> (w1640:u32[])
                    n1034 = property on="Saved AOD Raster Scan Parameter Sets" class="Arr (strict)"("Index Values"=w1640) -> ()  [unwired: 2 in, 2 out]
                    n1035 = property on="Trap Delta (MHz)" class="DigNum (strict)"("Val(Sgnl)"="Offset 1 Start (MHz)") -> ()  [unwired: 2 in, 2 out]
                  }
                  frame #1 {
                    n1036 = Wait (ms)(milliseconds to wait=u32 200) -> ()  [unwired: 1 out]
                  }
                  frame #2 {
                    n1037 = property on="Load parameters" class="Bool (strict)"("Val(Sgnl)"=TRUE ("Value (Signaling)")) -> ()  [unwired: 2 in, 2 out]
                  }
                  frame #3 {
                    n1038 = Wait (ms)(milliseconds to wait=u32 200) -> ()  [unwired: 1 out]
                  }
                  frame #4 {
                    n1039 = property on="Trap Raster Scan" class="Bool (strict)"("Val(Sgnl)"=TRUE ("Value (Signaling)")) -> ()  [unwired: 2 in, 2 out]
                  }
                  frame #5 {
                    n1040 = Wait (ms)(milliseconds to wait=u32 2000) -> ()  [unwired: 1 out]
                  }
                  frame #6 {
                    n1041 = while {
                      stop <- w1653 stop-if-true
                      n1042 = local read "Raster Scanning..."() -> (w1655:bool)
                      n1043 = local read "Saving..."() -> (w1651:bool)
                      n1044 = Wait (ms)(milliseconds to wait=u32 100) -> ()  [unwired: 1 out]
                      n1045 = Not(x=w1651) -> (.not. x?=w1650:bool)
                      n1046 = Not(x=w1655) -> (.not. x?=w1652:bool)
                      n1047 = And(x=w1652, y=w1650) -> (x .and. y?=w1653:bool)
                    }
                  }
                  frame #7 {
                    n1048 = property on="Trap Delta (MHz)" class="DigNum (strict)"("Val(Sgnl)"=w1656) -> ()  [unwired: 2 in, 2 out]
                  }
                }
              }
            }
          }
          frame #6 {
            n1049 = local read "Save ave N"() -> (w1657:dbl)
            n1050 = case shown="True" "W/ Offset 2" {
              tunnel: w1658 -> [_ w1664]
              tunnel: w1657 -> [_ w1663]
              frame False {
                n1051 = Multiply(x="Cal read wait (s)", y=u32 1000 ("milliseconds to wait")) -> (x*y=w1661:u32)
                n1052 = Wait (ms)(milliseconds to wait=w1661) -> ()  [unwired: 1 out]
              }
              frame True {
                n1053 = stacked-sequence {
                  tunnel: w1664 -> [_ _ _ _ _ _ _ _ _ w1685 _ _]
                  tunnel: w1663 -> [_ _ _ _ _ _ _ _ _ w1683 _ _]
                  frame #0 {
                    n1054 = property on="Save ave N" class="DigNum (strict)"("Val(Sgnl)"=1.0 ("Value (Signaling)")) -> ()  [unwired: 2 in, 2 out]
                  }
                  frame #1 {
                    n1055 = Wait (ms)(milliseconds to wait=u32 500) -> ()  [unwired: 1 out]
                  }
                  frame #2 {
                    n1056 = property on="Trap Delta (MHz)" class="DigNum (strict)"("Val(Sgnl)"="Offset 2 Start (MHz)") -> ()  [unwired: 2 in, 2 out]
                    n1057 = Replace Array Subset(array=u32[] [0] ("Index Values"), new element="Offset 2 Set", index=0) -> (w1669:u32[])
                    n1058 = property on="Saved AOD Raster Scan Parameter Sets" class="Arr (strict)"("Index Values"=w1669) -> ()  [unwired: 2 in, 2 out]
                  }
                  frame #3 {
                    n1059 = Wait (ms)(milliseconds to wait=u32 500) -> ()  [unwired: 1 out]
                  }
                  frame #4 {
                    n1060 = property on="Load parameters" class="Bool (strict)"("Val(Sgnl)"=TRUE ("Value (Signaling)")) -> ()  [unwired: 2 in, 2 out]
                  }
                  frame #5 {
                    n1061 = Wait (ms)(milliseconds to wait=u32 500) -> ()  [unwired: 1 out]
                  }
                  frame #6 {
                    n1062 = property on="Trap Raster Scan" class="Bool (strict)"("Val(Sgnl)"=TRUE ("Value (Signaling)")) -> ()  [unwired: 2 in, 2 out]
                  }
                  frame #7 {
                    n1063 = Wait (ms)(milliseconds to wait=u32 2000) -> ()  [unwired: 1 out]
                  }
                  frame #8 {
                    n1064 = while {
                      stop <- w1678 stop-if-true
                      n1065 = local read "Raster Scanning..."() -> (w1681:bool)
                      n1066 = local read "Saving..."() -> (w1679:bool)
                      n1067 = Wait (ms)(milliseconds to wait=u32 100) -> ()  [unwired: 1 out]
                      n1068 = Not(x=w1679) -> (.not. x?=w1677:bool)
                      n1069 = Not(x=w1681) -> (.not. x?=w1680:bool)
                      n1070 = And(x=w1680, y=w1677) -> (x .and. y?=w1678:bool)
                    }
                  }
                  frame #9 {
                    n1071 = property on="Trap Delta (MHz)" class="DigNum (strict)"("Val(Sgnl)"=w1685) -> ()  [unwired: 2 in, 2 out]
                    n1072 = property on="Saved AOD Raster Scan Parameter Sets" class="Arr (strict)"("Index Values"=u32[] [0]) -> ()  [unwired: 2 in, 2 out]
                    n1073 = property on="Save ave N" class="DigNum (strict)"("Val(Sgnl)"=w1683) -> ()  [unwired: 2 in, 2 out]
                  }
                  frame #10 {
                    n1074 = Wait (ms)(milliseconds to wait=u32 500) -> ()  [unwired: 1 out]
                  }
                  frame #11 {
                    n1075 = property on="Load parameters" class="Bool (strict)"("Val(Sgnl)"=TRUE ("Value (Signaling)")) -> ()  [unwired: 2 in, 2 out]
                  }
                }
              }
            }
          }
          frame #7 {
            n1076 = property on="Read Cal" class="Bool (strict)"("Val(Sgnl)"=TRUE ("Value (Signaling)")) -> ()  [unwired: 2 in, 2 out]
          }
          frame #8 {
            n1077 = Wait (ms)(milliseconds to wait=u32 500) -> ()  [unwired: 1 out]
          }
          frame #9 {
            n1078 = property on="Fish for Tether" class="Bool (strict)"("Val(Sgnl)"=FALSE ("Value (Signaling)")) -> ()  [unwired: 2 in, 2 out]
          }
        }
      }
      event "Dump Beads": Value Change {
        # "SCRIPT TO REMOVE BOTH BEADS FROM THE TRAPS. TURNS ON LIGHT WHICH INDICATES THAT STAGE IS MOVING. THEN STOPS SAVING DATA. \nSETS Sample Channel Flow TO TRUE. STOPS INTERLACING GREEN FLUORESCENCE. TURNS OFF Tether INDICATOR BECAUSE WE ARE THROWING IT\nAWAY. SHUTS OFF TRAP POSITION FEEDBACK."
        n1079 = event-data() -> ()  [unwired: 1 in, 5 out]
        n1080 = flat-sequence {
          frame #0 {
            w1692 = FALSE ("Fl. Triggered...")
            w1693 = TRUE ("Stage Moving")
            n1081 = local read "Saving..."() -> (w1694:bool)
            n1082 = local write "Fl. Triggered..."(w1692) -> ()
            n1083 = local write "Stage Moving"(w1693) -> ()
            n1084 = local write "Tether"(w1692) -> ()
            n1085 = property on="Green Laser ON/Interlacing" class="Bool (strict)"("Val(Sgnl)"=w1692) -> ()  [unwired: 2 in, 2 out]
            n1086 = property on="Trap Pos. FB ON" class="Bool (strict)"("Val(Sgnl)"=w1692) -> ()  [unwired: 2 in, 2 out]
            n1087 = property on="Inject Bottom" class="Bool (strict)"("Val(Sgnl)"=w1693) -> ()  [unwired: 2 in, 2 out]
            n1088 = local write "Stop Saving"(w1694) -> ()
          }
          frame #1 {
            w1695 = FALSE ("Value (Signaling)")
            # "TURNS TRAPS OFF SO THAT\nBEADS REMAIN AT DUMP \nBEADS POSITION"
            n1089 = property on="Trap 1 (ON/OFF)" class="Bool (strict)"("Val(Sgnl)"=w1695) -> ()  [unwired: 2 in, 2 out]
            n1090 = property on="Trap 2 (ON/OFF)" class="Bool (strict)"("Val(Sgnl)"=w1695) -> ()  [unwired: 2 in, 2 out]
            n1091 = call <vilib>:"Beep.vi"() -> ()  [unwired: 3 in, 9 out]
          }
          frame #2 {
            n1092 = property on="Goto Bottom (F7)" class="Bool (strict)"("Val(Sgnl)"=TRUE ("Value (Signaling)")) -> ()  [unwired: 2 in, 2 out]
          }
          frame #3 {
            n1093 = Wait (ms)(milliseconds to wait=u32 8000) -> ()  [unwired: 1 out]
          }
          frame #4 {
            n1094 = property on="Trap Delta (MHz)" class="DigNum (strict)"("Val(Sgnl)"=20.0 ("Value (Signaling)")) -> ()  [unwired: 2 in, 2 out]
          }
          frame #5 {
            n1095 = property on="Trap 2 (ON/OFF)" class="Bool (strict)"("Val(Sgnl)"=TRUE ("Value (Signaling)")) -> ()  [unwired: 2 in, 2 out]
          }
          frame #6 {
            n1096 = property on="Inject Bottom" class="Bool (strict)"("Val(Sgnl)"=FALSE ("Value (Signaling)")) -> ()  [unwired: 2 in, 2 out]
          }
        }
      }
      event "Dip for Protein": Value Change {
        n1097 = event-data() -> ()  [unwired: 1 in, 5 out]
        n1098 = flat-sequence {
          frame #0 {
            n1099 = case shown="True" "Move Trap Before?" {
              frame False {
              }
              frame True {
                n1100 = property on="Trap Delta (MHz)" class="DigNum (strict)"("Val(Sgnl)"="Dip Trap Delta 1 (MHz)") -> ()  [unwired: 2 in, 2 out]
              }
            }
          }
          frame #1 {
            n1101 = Multiply(x="Duration (s)", y=1000.0) -> (x*y=w1704:dbl)
            n1102 = Wait (ms)(milliseconds to wait=w1704) -> ()  [unwired: 1 out]
          }
          frame #2 {
